vi "Controller Write PID Parameters.vi"(8 "Error In":errorcluster, 9 "Automatic Mode?":bool, 10 "Ti":dbl, 11 "Ts":dbl) -> (0 "Error Out":errorcluster)   [LabVIEW 2011, in "Controller VIs.lvlib"]
uses:
  Controller VIs.lvlib
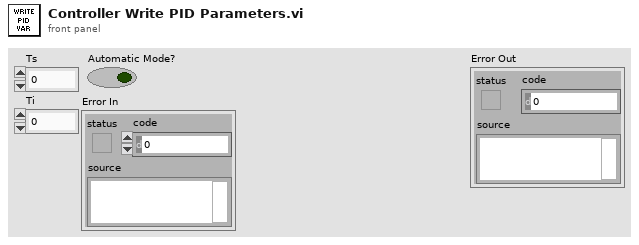
[diagram p1: front panel]
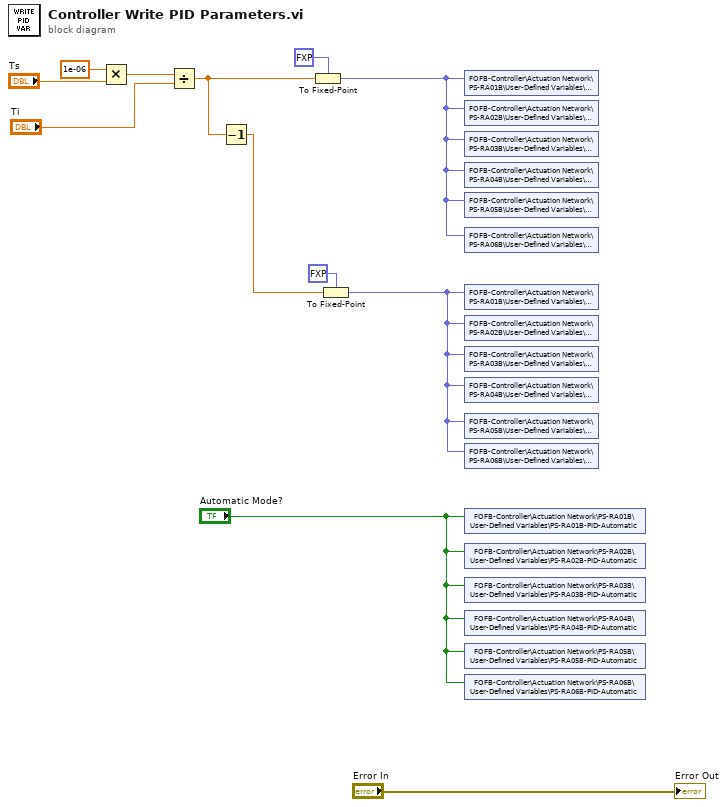
[diagram p0: block diagram]
diagram:
  n1 = Multiply(x=1e-06, y="Ts") -> (x*y=w7:dbl)
  n2 = Divide(x=w7, y="Ti") -> (x/y=w10:dbl)
  n3 = Decrement(x=w10) -> (x-1=w6:dbl)
  n4 = To Fixed-Point(fixed-point type=fxp<+/-,18,1> 0.0 ("PS-RA01B-PID-I1"), number=w10) -> (fixed-point=w4:fxp<+/-,18,1>)
  n5 = To Fixed-Point(fixed-point type=fxp<+/-,18,2> 0.0 ("PS-RA01B-PID-I2"), number=w6) -> (fixed-point=w2:fxp<+/-,18,2>)
  n6 = shared-variable "FOFB-Controller\\Actuation Network\\PS-RA01B\\User-Defined Variables\\PS-RA01B-PID-I1"(w4) -> ()  [unwired: 1 in, 1 out]
  n7 = shared-variable "FOFB-Controller\\Actuation Network\\PS-RA02B\\User-Defined Variables\\PS-RA02B-PID-I1"(w4) -> ()  [unwired: 1 in, 1 out]
  n8 = shared-variable "FOFB-Controller\\Actuation Network\\PS-RA03B\\User-Defined Variables\\PS-RA03B-PID-I1"(w4) -> ()  [unwired: 1 in, 1 out]
  n9 = shared-variable "FOFB-Controller\\Actuation Network\\PS-RA04B\\User-Defined Variables\\PS-RA04B-PID-I1"(w4) -> ()  [unwired: 1 in, 1 out]
  n10 = shared-variable "FOFB-Controller\\Actuation Network\\PS-RA05B\\User-Defined Variables\\PS-RA05B-PID-I1"(w4) -> ()  [unwired: 1 in, 1 out]
  n11 = shared-variable "FOFB-Controller\\Actuation Network\\PS-RA06B\\User-Defined Variables\\PS-RA06B-PID-I1"(w4) -> ()  [unwired: 1 in, 1 out]
  n12 = shared-variable "FOFB-Controller\\Actuation Network\\PS-RA01B\\User-Defined Variables\\PS-RA01B-PID-I2"(w2) -> ()  [unwired: 1 in, 1 out]
  n13 = shared-variable "FOFB-Controller\\Actuation Network\\PS-RA02B\\User-Defined Variables\\PS-RA02B-PID-I2"(w2) -> ()  [unwired: 1 in, 1 out]
  n14 = shared-variable "FOFB-Controller\\Actuation Network\\PS-RA03B\\User-Defined Variables\\PS-RA03B-PID-I2"(w2) -> ()  [unwired: 1 in, 1 out]
  n15 = shared-variable "FOFB-Controller\\Actuation Network\\PS-RA04B\\User-Defined Variables\\PS-RA04B-PID-I2"(w2) -> ()  [unwired: 1 in, 1 out]
  n16 = shared-variable "FOFB-Controller\\Actuation Network\\PS-RA05B\\User-Defined Variables\\PS-RA05B-PID-I2"(w2) -> ()  [unwired: 1 in, 1 out]
  n17 = shared-variable "FOFB-Controller\\Actuation Network\\PS-RA06B\\User-Defined Variables\\PS-RA06B-PID-I2"(w2) -> ()  [unwired: 1 in, 1 out]
  n18 = shared-variable "FOFB-Controller\\Actuation Network\\PS-RA01B\\User-Defined Variables\\PS-RA01B-PID-Automatic"("Automatic Mode?") -> ()  [unwired: 1 in, 1 out]
  n19 = shared-variable "FOFB-Controller\\Actuation Network\\PS-RA02B\\User-Defined Variables\\PS-RA02B-PID-Automatic"("Automatic Mode?") -> ()  [unwired: 1 in, 1 out]
  n20 = shared-variable "FOFB-Controller\\Actuation Network\\PS-RA03B\\User-Defined Variables\\PS-RA03B-PID-Automatic"("Automatic Mode?") -> ()  [unwired: 1 in, 1 out]
  n21 = shared-variable "FOFB-Controller\\Actuation Network\\PS-RA04B\\User-Defined Variables\\PS-RA04B-PID-Automatic"("Automatic Mode?") -> ()  [unwired: 1 in, 1 out]
  n22 = shared-variable "FOFB-Controller\\Actuation Network\\PS-RA05B\\User-Defined Variables\\PS-RA05B-PID-Automatic"("Automatic Mode?") -> ()  [unwired: 1 in, 1 out]
  n23 = shared-variable "FOFB-Controller\\Actuation Network\\PS-RA06B\\User-Defined Variables\\PS-RA06B-PID-Automatic"("Automatic Mode?") -> ()  [unwired: 1 in, 1 out]
  "Error Out" <- "Error In"
